vi "Address Space Size.vi"(2 "niUSRP DSP v2 FPGA":refnum<class "niUSRP Rx DSP v2 FPGA.lvclass">) -> (6 "size":u32)   [LabVIEW 2025, in "niUSRP Rx DSP v2 FPGA.lvclass"]
uses:
  niUSRP Rx DSP v2 FPGA.lvclass
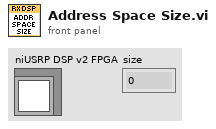
[diagram p1: front panel]
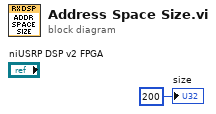
[diagram p0: block diagram]
diagram:
  "size" <- u32 200 ("size")
